vi "getMensagem.vi"(3 "Mensagem in":refnum<class "Mensagem.lvclass">) -> (0 "mensagem":string, 1 "Mensagem out":refnum<class "Mensagem.lvclass">)   [LabVIEW 2015, in "Mensagem.lvclass"]
uses:
  Mensagem.lvclass
  Mensagem.lvclass/Mensagem.ctl
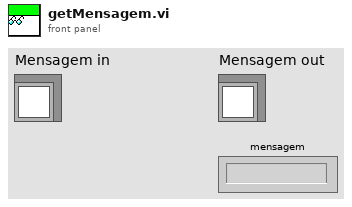
[diagram p1: front panel]
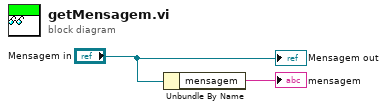
[diagram p0: block diagram]
diagram:
  n1 = Unbundle By Name("Mensagem in") -> ("mensagem"=→"mensagem":string)
  "Mensagem out" <- "Mensagem in"
